vi "UTC Offset to Seconds.vi"(11 "UTC Offset String":string) -> (1 "Valid?":bool, 2 "Offset (s)":ext, 3 "UTC Offset":T1=enum."UTC+00:00")   [LabVIEW 2021]
uses:
  UTC Offsets -- enum.ctl
  <vilib>/regexp/Match Regular Expression.xnode
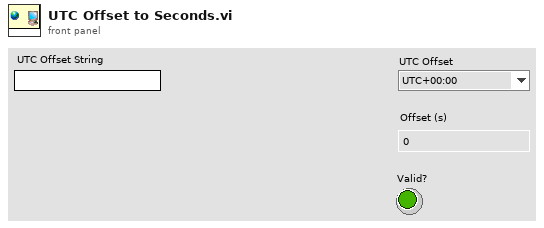
[diagram p1: front panel]
types:
  T1 = typedef "UTC Offsets -- enum.ctl" = enum16{"UTC-12:00", "UTC-11:00", "UTC-10:00", "UTC-09:30", "UTC-09:00", "UTC-08:00", "UTC-07:00", "UTC-06:00", "UTC-05:00", "UTC-04:00", "UTC-03:30", "UTC-03:00", "UTC-02:00", "UTC-01:00", "UTC-00:00", "UTC+00:00", "UTC+01:00", "UTC+02:00", "UTC+03:00", "UTC+03:30", "UTC+04:00", "UTC+04:30", "UTC+05:00", "UTC+05:30", "UTC+05:45", "UTC+06:00", "UTC+06:30", "UTC+07:00", "UTC+08:00", "UTC+08:45", "UTC+09:00", "UTC+09:30", "UTC+10:00", "UTC+10:30", "UTC+11:00", "UTC+12:00", "UTC+12:45", "UTC+13:00", "UTC+14:00"}
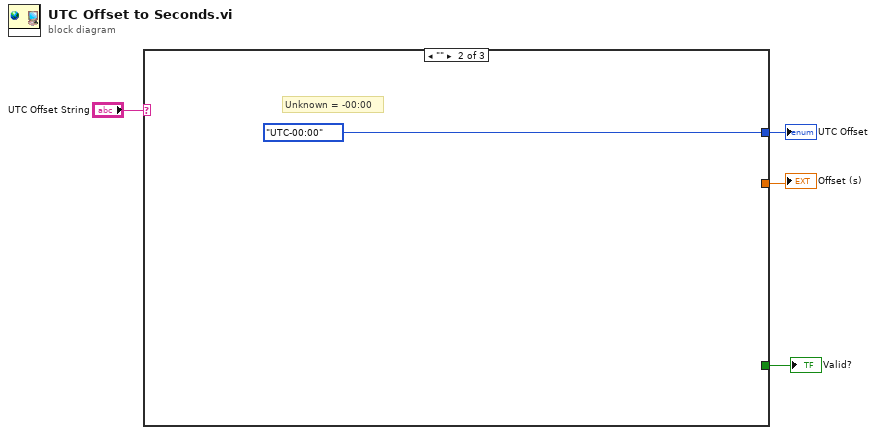
[diagram p0: block diagram]
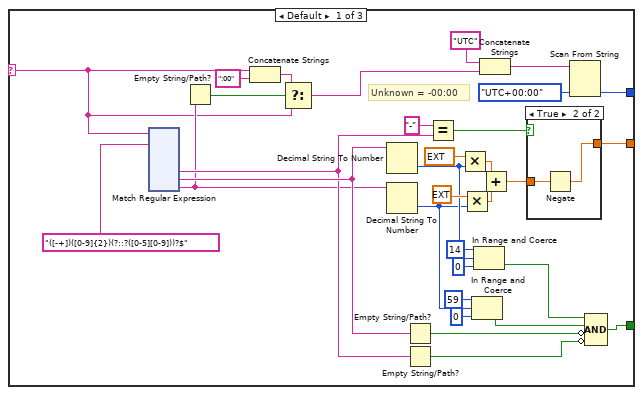
[diagram p2: hidden frame]
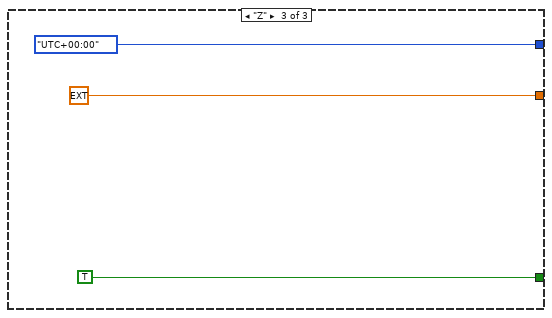
[diagram p4: hidden frame]
diagram:
  n1 = case shown="\"\"" "UTC Offset String" {
    selector: "UTC Offset String" -> [w6 _ _]
    tunnel: [w35 UTC_Offsets_--_enum."UTC-00:00" ("UTC Time Offset") UTC_Offsets_--_enum."UTC+00:00" ("UTC Time Offset")] -> w4
    tunnel: [w25 _ ext 0.0] -> w3
    tunnel: [w21 _ TRUE] -> w2
    frame Default {
      # "Unknown = -00:00"
      n2 = xnode "Match Regular Expression"("input string"=w6, "regular expression"="([-+])([0-9]{2})(?::?([0-5][0-9]))?$") -> ("submatch 1"=w23:string, "submatch 2"=w24:string, "submatch 3"=w10:string)  [unwired: 4 in, 5 out]
      n3 = Empty String/Path?(string/path=w10) -> (empty?=w9:bool)
      n4 = Concatenate Strings(w6, ":00" ("string")) -> (w8:string)
      n5 = Select(t=w8, s=w9, f=w6) -> (s? t:f=w7:string)
      n6 = Decimal String To Number(string=w24) -> (number=w20:i32)  [unwired: 2 in, 1 out]
      n7 = Decimal String To Number(string=w10) -> (number=w14:i32)  [unwired: 2 in, 1 out]
      n8 = Empty String/Path?(string/path=w24) -> (empty?=w22:bool)
      n9 = Empty String/Path?(string/path=w23) -> (empty?=w11:bool)
      n10 = Equal?(x="-" ("y"), y=w23) -> (x = y?=w26:bool)
      n11 = Multiply(x=ext 3600.0, y=w20) -> (x*y=w30:ext)
      n12 = Multiply(x=ext 60.0, y=w14) -> (x*y=w29:ext)
      n13 = In Range and Coerce(upper limit=59, x=w14, lower limit=0) -> (In Range?=w13:bool)  [unwired: 1 out]
      n14 = In Range and Coerce(upper limit=14, x=w20, lower limit=0) -> (In Range?=w17:bool)  [unwired: 1 out]
      n15 = Concatenate Strings("UTC" ("format string"), w7) -> (w34:string)
      n16 = Add(x=w30, y=w29) -> (x+y=w28:ext)
      n17 = case shown="True" w26 {
        tunnel: w28 -> [w158 w160]
        tunnel: [w158 w159] -> w25
        frame False {
        }
        frame True {
          n18 = Negate(x=w160) -> (-x=w159:ext)
        }
      }
      n19 = Scan From String(input string=w34, default 1=UTC_Offsets_--_enum."UTC+00:00" ("UTC Time Offset")) -> (output 1=w35:T1)  [unwired: 3 in, 3 out]
      n20 = Compound Arithmetic op=AND(w17, w13, invert w22, invert w11) -> (w21:bool)
    }
    frame "" {
      # "Unknown = -00:00"
    }
    frame "Z" {
    }
  }
  "UTC Offset" <- w4
  "Offset (s)" <- w3
  "Valid?" <- w2
